vi "analyze voltage.vi"(0 "display queues":T3, 3 "time range (s)":dbl=2.2 format="%#_13g", 4 "gain":dbl=1.0, 5 "volt slope":bool, 7 "error in":errorcluster, 8 "trigger":bool, 9 "hysteresis":dbl=0.1 format="%#_13g", 10 "disk queues":T3) -> (20 "crossing stats":T2, 23 "voltage axes":T1, 24 "voltage graphs":cluster{dbl[], dbl[]}[](array[cluster]), 27 "error out":errorcluster)   [LabVIEW 2017]
uses:
  typedefs/queue cluster.ctl
  typedefs/reading queue.ctl
  typedefs/reading.ctl
  typedefs/readingType.ctl
  typedefs/reading 1 queue.ctl
  typedefs/reading1.ctl
  popup panels/control panel globals.vi
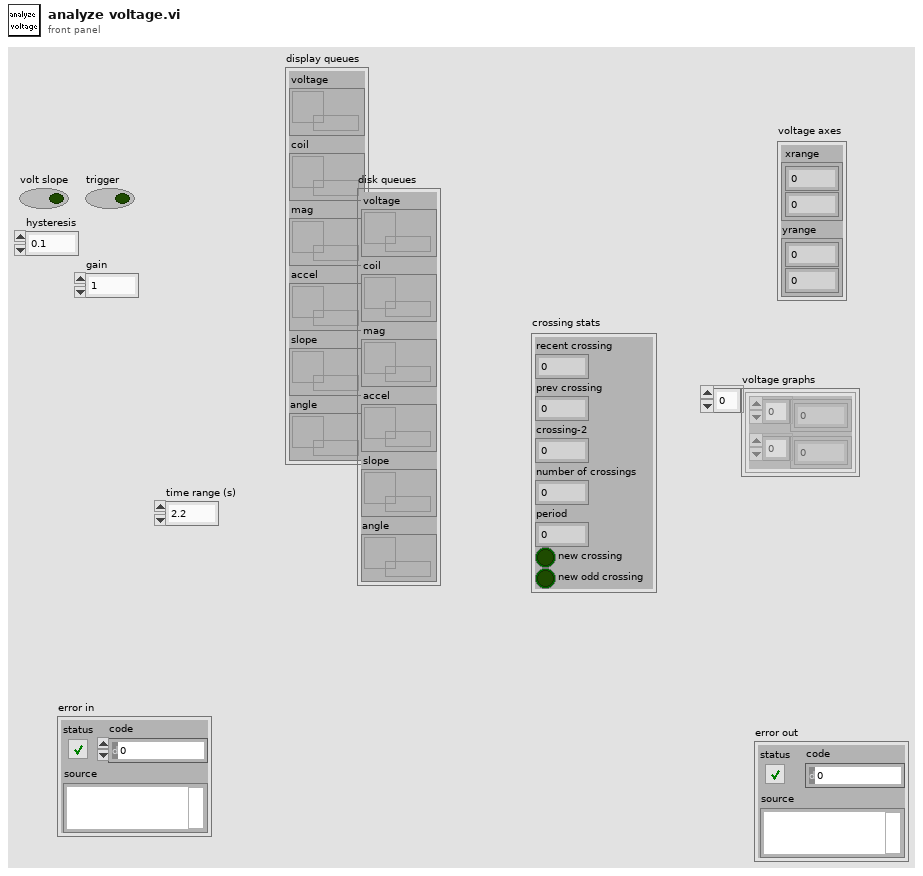
[diagram p1: front panel]
types:
  T1 = cluster{" xrange":cluster{dbl, dbl}, "yrange":cluster{dbl, dbl}}
  T2 = cluster{"recent crossing":dbl, "prev crossing":dbl, "crossing-2":dbl, "number of crossings":i32, "period":dbl, "new crossing":bool, "new odd crossing":bool}
  T3 = typedef "queue cluster.ctl" = cluster{"voltage":T4, "coil":T4, "mag":T4, "accel":T4, "slope":T5, "angle":T4}
  T4 = typedef "reading queue.ctl" = refnum<queue>
  T5 = typedef "reading 1 queue.ctl" = refnum<queue>
  T6 = typedef "reading.ctl" = cluster{"reading type":T7, "time":fxp<+,48,48>, "x":sgl, "y":sgl, "z":sgl, "XSUM":u8}
  T7 = typedef "readingType.ctl" = enum8{"SYNC", "DETVAL", "COILI", "MAGVEC", "ACCVEC"}
  T8 = cluster{"tx":cluster{dbl[], sgl[]}, "ty":cluster{dbl[], sgl[]}, "tz":cluster{dbl[], sgl[]}, "xy":cluster{sgl[], sgl[]}}
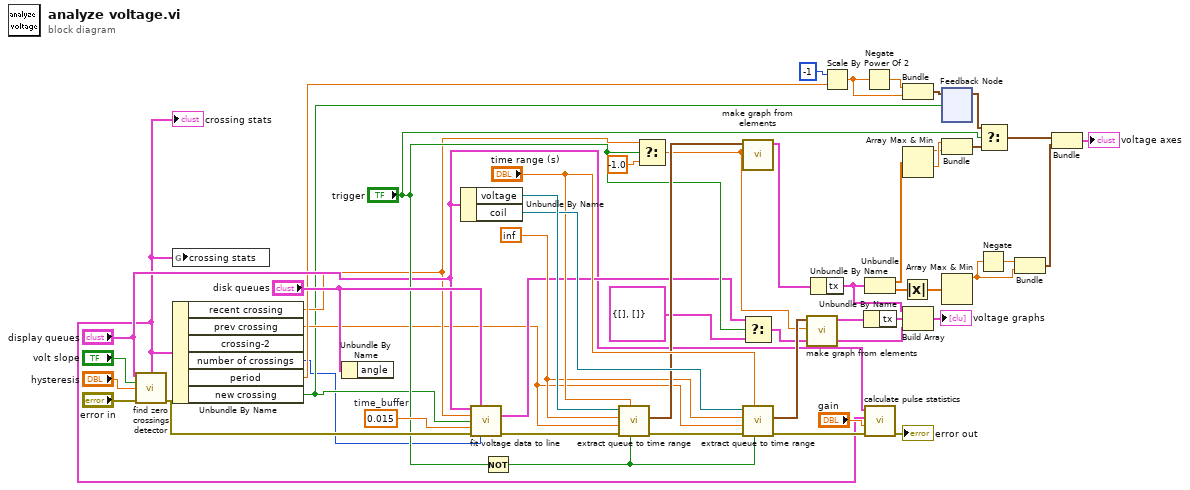
[diagram p0: block diagram]
diagram:
  w28 = inf
  w49 = 0.015  # time_buffer
  n1 = call "find zero crossings detector.vi"("display queues"="display queues", "slope"="volt slope", "hysteresis"="hysteresis", "error in (no error)"="error in") -> ("crossing stats"=w2:T2, "error out"=w48:errorcluster)  [unwired: 4 in, 6 out]
  "crossing stats" <- w2
  n2 = global write "control panel globals.vi" "crossing stats"(w2) -> ()
  n3 = Unbundle By Name(w2) -> ("recent crossing"=w12:dbl, "prev crossing"=w11:dbl, "number of crossings"=w3:i32, "period"=w13:dbl, "new crossing"=w7:bool)  [unwired: 1 out]
  n4 = Unbundle By Name("disk queues") -> ()  [unwired: 1 out]
  n5 = Unbundle By Name("display queues") -> ("voltage"=w39:T4, "coil"=w38:T4)
  n6 = call "fit voltage data to line.vi"("display queues"="display queues", "disk queues"="disk queues", "crossing time"=w12, "new odd crossing"=w7, "time_buffer"=w49, "error in (no error)"=w48, "crossing number"=w3) -> ("graph"=w27:cluster{dbl[], "Best Linear Fit":dbl[]}, "error out"=w1:errorcluster)  [unwired: 6 in, 1 out]
  n7 = Not(x="trigger") -> (.not. x?=w36:bool)
  n8 = call "extract queue to time range.vi"("most recent?"=w36, "recent interval"="time range (s)", "error in (no error)"=w1, "t0"=w11, "t1"=w28, "queue"=w39) -> ("error out"=w19:errorcluster, "extracted data"=w35:T6[])  [unwired: 4 in]
  n9 = Select(t=w12, s="trigger", f=-1.0) -> (s? t:f=w32:dbl)
  n10 = call "make graph from elements.vi"("toffset"=w32, "elements"=w35) -> ("graphs"=w22:T8)  [unwired: 8 in, 1 out]
  n11 = Select(t=w27, s="trigger", f=cluster{dbl[], dbl[]} {[], []} ("element")) -> (s? t:f=w26:cluster{dbl[], "Best Linear Fit":dbl[]})
  n12 = call "extract queue to time range.vi"("most recent?"=w36, "recent interval"="time range (s)", "error in (no error)"=w19, "t0"=w11, "t1"=w28, "queue"=w38) -> ("error out"=w20:errorcluster, "extracted data"=w33:T6[])  [unwired: 4 in]
  n13 = call "make graph from elements.vi"("toffset"=w32, "elements"=w33) -> ("graphs"=w21:T8)  [unwired: 8 in, 1 out]
  n14 = Unbundle By Name(w22) -> ("tx"=w17:cluster{dbl[], sgl[]})
  n15 = Scale By Power Of 2(n=i16 -1, x=w13) -> (x*2^n=w5:dbl)
  n16 = Negate(x=w5) -> (-x=w18:dbl)
  n17 = Unbundle By Name(w21) -> ("tx"=w31:cluster{dbl[], sgl[]})
  n18 = Unbundle(w17) -> (w16:dbl[], w15:sgl[])
  n19 = call "calculate pulse statistics.vi"("error in (no error)"=w20, "gain"="gain", "crossing stats"=w2, "display queues"="display queues") -> ("error out"=→"error out":errorcluster)  [unwired: 7 in]
  n20 = Absolute Value(x=w15) -> (abs(x)=w6:sgl[])
  n21 = Bundle(w18, w5) -> (w50:cluster{dbl, dbl})  [unwired: 1 in]
  n22 = Array Max & Min(array=w16) -> (max value=w42:dbl, min value=w43:dbl)  [unwired: 2 out]
  n23 = Build Array(w17, w31, w26) -> (→"voltage graphs":cluster{dbl[], "Best Linear Fit":dbl[]}[])
  n24 = feedback-in #1(w50, w7) -> ()
  n25 = feedback #1() -> (w44:cluster{dbl, dbl})  [unwired: 1 in]
  n26 = Bundle(w43, w42) -> (w41:cluster{dbl, dbl})  [unwired: 1 in]
  n27 = Array Max & Min(array=w6) -> (max value=w45:sgl)  [unwired: 3 out]
  n28 = Negate(x=w45) -> (-x=w46:sgl)
  n29 = Select(t=w44, s="trigger", f=w41) -> (s? t:f=w9:cluster{dbl, dbl})
  n30 = Bundle(w46, w45) -> (w10:cluster{sgl, sgl})  [unwired: 1 in]
  n31 = Bundle(w9, w10) -> (→"voltage axes":cluster{cluster{dbl, dbl}, cluster{sgl, sgl}})  [unwired: 1 in]
